vi "FID mit Propan Linearisieren.vi"(10 "Werte":string[](array[string])) -> (2 "Werte":string[](array[string]))   [LabVIEW 2020, in "ABB-EL3000.lvlib" / "FID.lvlib" / "FID Kalibrierung.lvlib"]
uses:
  FID Kalibrierung.lvlib
  Aktionen FID Kal Komponente.ctl
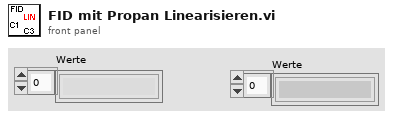
[diagram p1: front panel]
types:
  T1 = typedef "ABB-EL3000.lvlib/FID.lvlib/FID Kalibrierung.lvlib/Aktionen FID Kal Komponente.ctl" = enum16{"lesen", "setzen", "laden", "speichern", "LIN"}
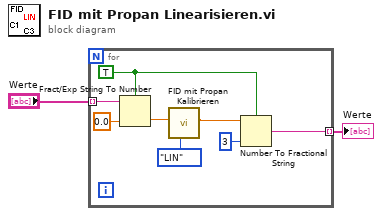
[diagram p0: block diagram]
diagram:
  n1 = for {
    tunnel: "Werte" -> [w10] mode=indexing
    tunnel: [w6] -> w1 mode=indexing
    w7 = TRUE ("Systemdezimalzeichen verwenden (T)")
    n2 = Fract/Exp String To Number(use system decimal point (T)=w7, string=w10, default (0 dbl)=sgl 0.0 ("Standard (0 DBL)")) -> (number=w5:sgl)  [unwired: 1 in, 1 out]
    n3 = call "FID mit Propan Kalibrieren.vi"("Aktionen"=Aktionen_FID_Kal_Komponente."LIN", "Wert"=w5) -> ("Wert"=w4:sgl)  [unwired: 8 in, 1 out]
    n4 = Number To Fractional String(use system decimal point (T)=w7, number=w4, precision (6)=i16 3 ("Genauigkeit (6)")) -> (F-format string=w6:string)  [unwired: 1 in]
  }
  "Werte" <- w1
